vi "Read HTS221 Temperature & Humidity.vi"(8 "error in (no error)":errorcluster, 11 "LINX-SenseHat in":refnum<class "LINX-SenseHat.lvclass">) -> (0 "error out":errorcluster, 2 "HTS221 Data":T1, 3 "LINX-SenseHat out":refnum<class "LINX-SenseHat.lvclass">)   [LabVIEW 2020, in "LINX-SenseHat.lvclass"]
doc: "Reads temperature/humidity data from the HTS221 sensor on the Sense Hat."
uses:
  LINX-SenseHat.lvclass
  HTS221 Data.ctl
  LINX-SenseHat.lvclass/LINX-SenseHat.ctl
  HTS221/HTS221.lvclass
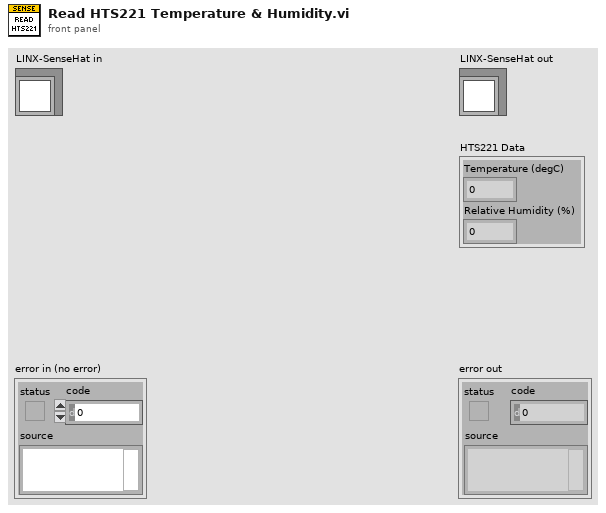
[diagram p1: front panel]
types:
  T1 = typedef "LINX-SenseHat.lvclass/HTS221 Data.ctl" = cluster{"Temperature (degC)":dbl, "Relative Humidity (%)":dbl}
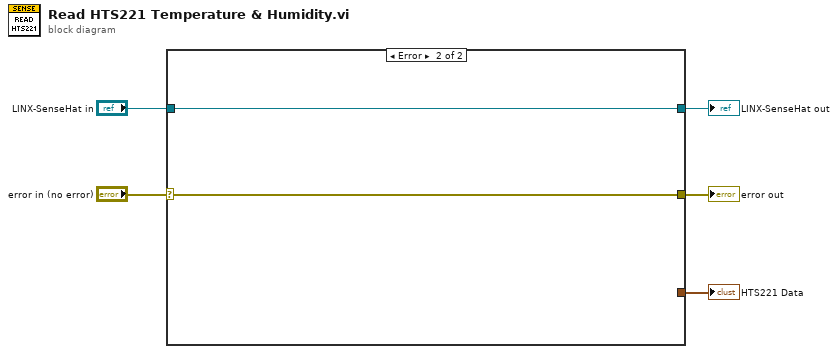
[diagram p0: block diagram]
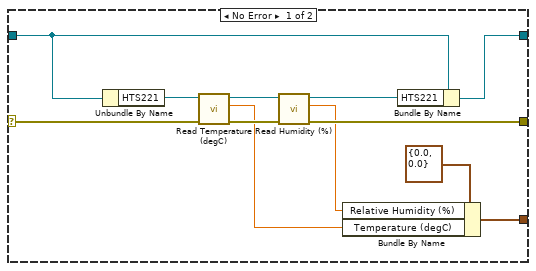
[diagram p2: hidden frame]
diagram:
  n1 = case shown="Error" "error in (no error)" {
    selector: "error in (no error)" -> [w15 w19]
    tunnel: [w10 w19] -> w4
    tunnel: [w16 w18] -> w2
    tunnel: "LINX-SenseHat in" -> [w17 w18]
    tunnel: [w6 _] -> w1
    frame No Error {
      n2 = Unbundle By Name(w17) -> ("HTS221"=w14:refnum<class "HTS221.lvclass">)
      n3 = call "Read Temperature (degC).vi"("error in (no error)"=w15, "HTS221 in"=w14) -> ("error out"=w13:errorcluster, "Temperature (degC)"=w9:dbl, "HTS221 out"=w12:refnum<class "HTS221.lvclass">)  [unwired: 7 in]
      n4 = call "Read Humidity (%).vi"("error in (no error)"=w13, "HTS221 in"=w12) -> ("error out"=w10:errorcluster, "Relative Humidity (%)"=w7:dbl, "HTS221 out"=w11:refnum<class "HTS221.lvclass">)  [unwired: 7 in]
      n5 = Bundle By Name(cluster=T1 {"Temperature (degC)"=0.0, "Relative Humidity (%)"=0.0}, "Relative Humidity (%)"=w7, "Temperature (degC)"=w9) -> (w6:T1)
      n6 = Bundle By Name(cluster=w17, "HTS221"=w11) -> (w16:refnum<class "LINX-SenseHat.lvclass">)
    }
    frame Error {
    }
  }
  "error out" <- w4
  "LINX-SenseHat out" <- w2
  "HTS221 Data" <- w1
